vi "optimise_BBO_position.vi"(0 "Laser Power Q":T2, 7 "Controls Cluster":T1 {"Initial Step Direction" items=["Negative", "Positive"]}, 11 "error in (no error)":errorcluster) -> (8 "Optimised BBO crystal position":i32, 15 "error out":errorcluster)   [LabVIEW 2023]
panel:
  in  "stop":bool
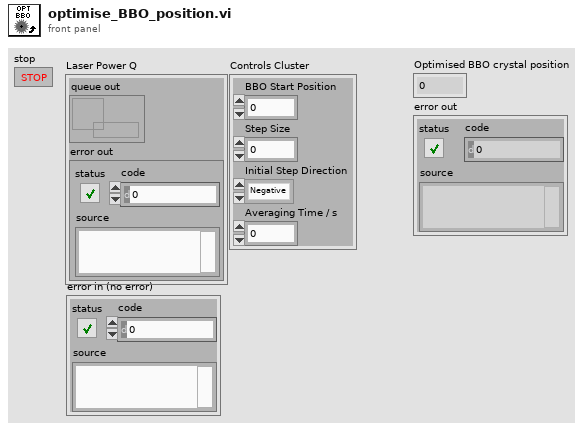
[diagram p1: front panel]
types:
  T1 = cluster{"BBO Start Position":i32, "Step Size":i32, "Initial Step Direction":u16, "Averaging Time / s ":u32}
  T2 = cluster{"queue out":refnum<queue>, "error out":errorcluster}
  T3 = cluster{"notifier out":refnum<notifier>, "error out":errorcluster}
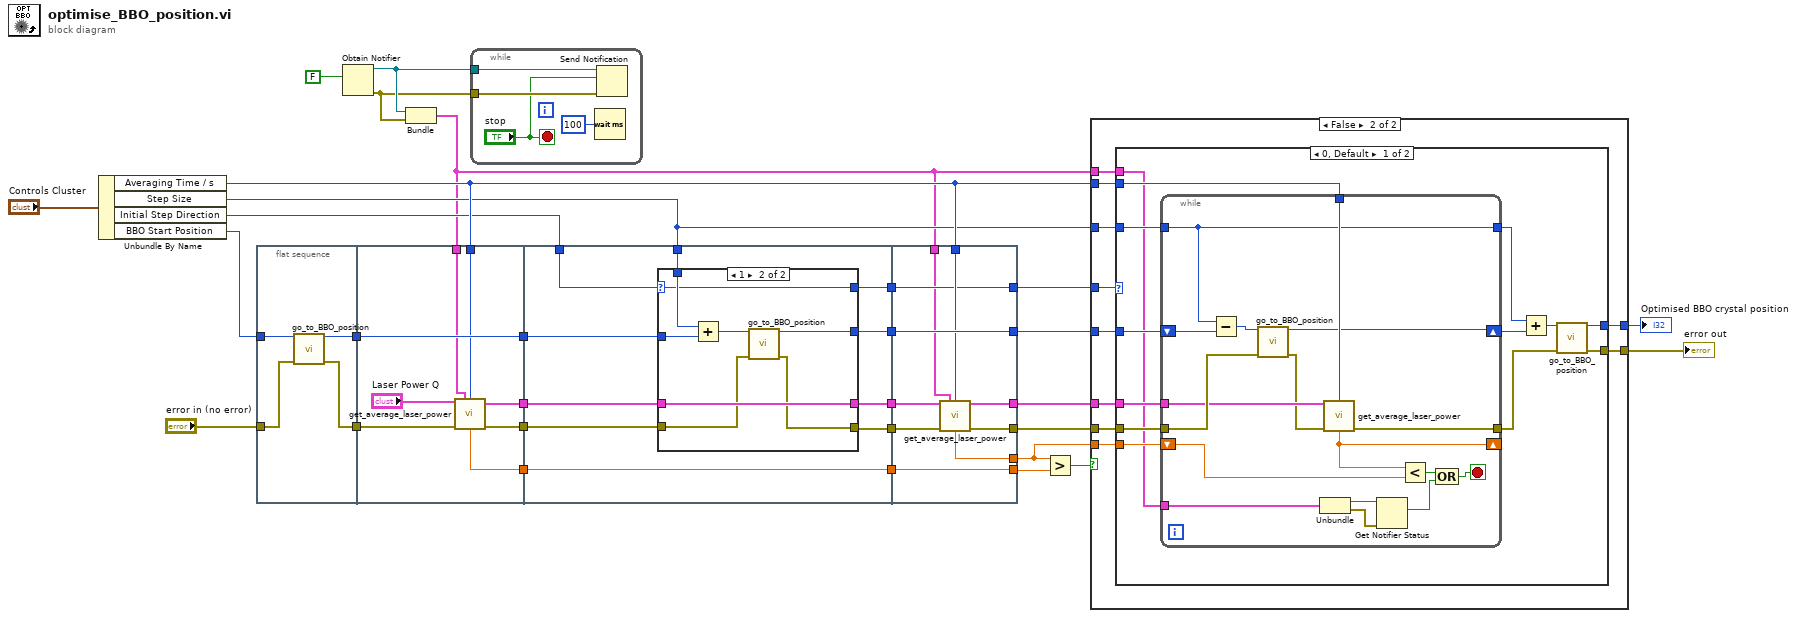
[diagram p0: block diagram]
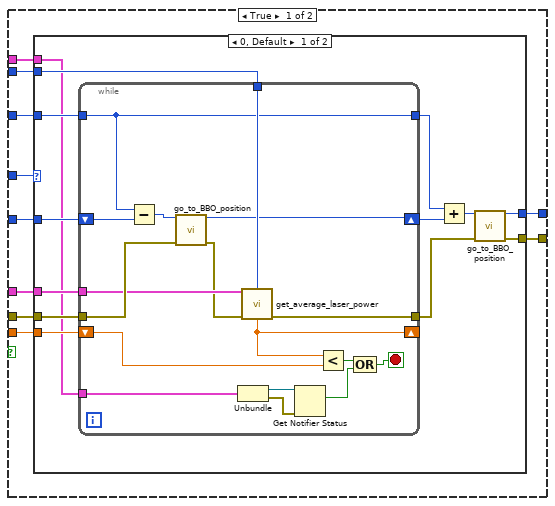
[diagram p2: hidden frame]
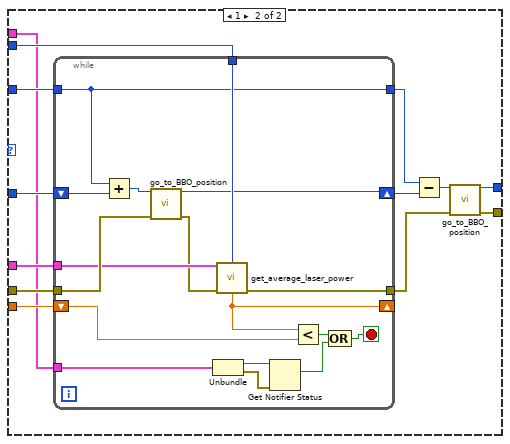
[diagram p3: hidden frame]
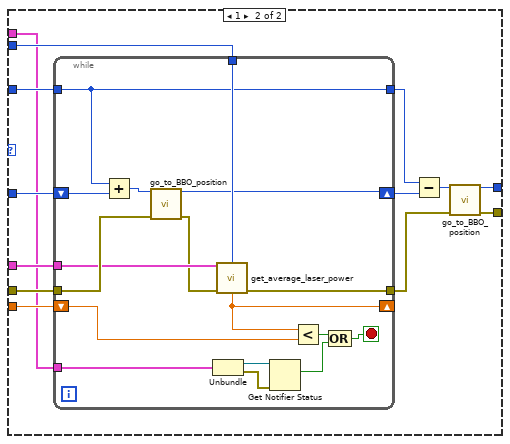
[diagram p4: hidden frame]
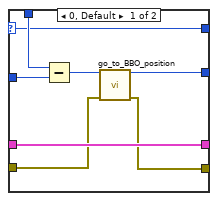
[diagram p5: hidden frame]
diagram:
  n1 = Unbundle By Name("Controls Cluster") -> ("Averaging Time / s"=w8:u32, "Step Size"=w6:i32, "Initial Step Direction"=w5:u16, "BBO Start Position"=w7:i32)
  n2 = flat-sequence {
    tunnel: w7 -> [w34]
    tunnel: "error in (no error)" -> [w33]
    tunnel: [w32] -> w29
    tunnel: [w31] -> w28
    tunnel: w29 -> [w42]
    tunnel: w28 -> [w37]
    tunnel: [w41] -> w27
    tunnel: [w40] -> w26
    tunnel: [w38] -> w25
    tunnel: [w37] -> w24
    tunnel: w8 -> [w36]
    tunnel: w1 -> [w35]
    tunnel: w27 -> [w50]
    tunnel: w26 -> [w45]
    tunnel: w25 -> [w51]
    tunnel: w24 -> [w49]
    tunnel: w6 -> [w52]
    tunnel: [w48] -> w23
    tunnel: [w47] -> w22
    tunnel: [w46] -> w21
    tunnel: [w45] -> w20
    tunnel: [w44] -> w14
    tunnel: w5 -> [w43]
    tunnel: w23 -> [w78]
    tunnel: w22 -> [w77]
    tunnel: w21 -> [w76]
    tunnel: w8 -> [w73]
    tunnel: w20 -> [w71]
    tunnel: [w78] -> w17
    tunnel: [w75] -> w16
    tunnel: [w74] -> w15
    tunnel: [w72] -> w12
    tunnel: [w71] -> w19
    tunnel: w14 -> [w70]
    tunnel: [w70] -> w13
    tunnel: w1 -> [w69]
    frame #0 {
      n3 = call "go_to_BBO_position.vi"("Set BBO crystal position"=w34, "error in (no error)"=w33) -> ("BBO crystal position"=w31:i32, "error out"=w32:errorcluster)  [unwired: 11 in, 1 out]
    }
    frame #1 {
      n4 = call "get_average_laser_power.vi"("Laser Power Q"="Laser Power Q", "Cancel Notifier"=w35, "Averaging Time /s"=w36, "Error in"=w42) -> ("Laser Power Q Out"=w38:T2, "Average Power / J"=w40:dbl, "Error out"=w41:errorcluster)  [unwired: 9 in]
    }
    frame #2 {
      n5 = case shown="1" w43 {
        selector: w43 -> [w53 w61]
        tunnel: w52 -> [w56 w64]
        tunnel: w51 -> [w60 w68]
        tunnel: [w60 w68] -> w47
        tunnel: w50 -> [w59 w67]
        tunnel: [w58 w66] -> w46
        tunnel: w49 -> [w55 w63]
        tunnel: [w54 w62] -> w48
        tunnel: [w53 w61] -> w44
        frame 0, Default {
          n6 = Subtract(x=w56, y=w55) -> (x-y=w57:i32)
          n7 = call "go_to_BBO_position.vi"("Set BBO crystal position"=w57, "error in (no error)"=w59) -> ("BBO crystal position"=w54:i32, "error out"=w58:errorcluster)  [unwired: 11 in, 1 out]
        }
        frame 1 {
          n8 = Add(x=w64, y=w63) -> (x+y=w65:i32)
          n9 = call "go_to_BBO_position.vi"("Set BBO crystal position"=w65, "error in (no error)"=w67) -> ("BBO crystal position"=w62:i32, "error out"=w66:errorcluster)  [unwired: 11 in, 1 out]
        }
      }
    }
    frame #3 {
      n10 = call "get_average_laser_power.vi"("Laser Power Q"=w77, "Cancel Notifier"=w69, "Averaging Time /s"=w73, "Error in"=w76) -> ("Laser Power Q Out"=w75:T2, "Average Power / J"=w72:dbl, "Error out"=w74:errorcluster)  [unwired: 9 in]
    }
  }
  n11 = Obtain Notifier(notification data type=FALSE ("stop")) -> (notifier out=w3:refnum<notifier>, error out=w2:errorcluster)  [unwired: 3 in, 1 out]
  n12 = Bundle("notifier out"=w3, "error out"=w2) -> (w1:T3)  [unwired: 1 in]
  n13 = while {
    tunnel: w3 -> [w81]
    tunnel: w2 -> [w80]
    stop <- "stop" stop-if-true
    n14 = Wait (ms)(milliseconds to wait=u32 100) -> ()  [unwired: 1 out]
    n15 = Send Notification(notification="stop", notifier=w81, error in (no error)=w80) -> ()  [unwired: 2 out]
  }
  n16 = Greater?(x=w12, y=w19) -> (0:w18:bool)
  n17 = case shown="False" w18 {
    tunnel: w17 -> [w91 w161]
    tunnel: w16 -> [w90 w160]
    tunnel: w15 -> [w89 w159]
    tunnel: w13 -> [w92 w162]
    tunnel: w6 -> [w88 w158]
    tunnel: w8 -> [w87 w157]
    tunnel: w12 -> [w86 w156]
    tunnel: [w85 w155] -> w11
    tunnel: [w84 w154] -> w10
    tunnel: w1 -> [w83 w153]
    frame True {
      n18 = case shown="0, Default" w92 {
        tunnel: w91 -> [w105 w135]
        tunnel: w90 -> [w104 w134]
        tunnel: w89 -> [w103 w133]
        tunnel: w88 -> [w102 w132]
        tunnel: w87 -> [w101 w131]
        tunnel: w86 -> [w100 w130]
        tunnel: [w95 w125] -> w85
        tunnel: [w94 w124] -> w84
        tunnel: w83 -> [w93 w123]
        frame 0, Default {
          n19 = while {
            tunnel: w104 -> [w119]
            tunnel: w103 -> [w122]
            tunnel: w102 -> [w112]
            tunnel: [w117] -> w96
            tunnel: w101 -> [w116]
            shift-right: [w115] -> w99
            shift-left: w105 -> [w120]
            shift-right: [w114] -> _
            shift-left: w100 -> [w113]
            tunnel: [w112] -> w98
            tunnel: w93 -> [w111]
            stop <- w108 stop-if-true
            n20 = Subtract(x=w112, y=w120) -> (x-y=w121:i32)
            n21 = call "go_to_BBO_position.vi"("Set BBO crystal position"=w121, "error in (no error)"=w122) -> ("BBO crystal position"=w115:i32, "error out"=w118:errorcluster)  [unwired: 11 in, 1 out]
            n22 = Unbundle(w111) -> ("notifier out"=w110:refnum<notifier>, "error out"=w109:errorcluster)
            n23 = call "get_average_laser_power.vi"("Laser Power Q"=w119, "Averaging Time /s"=w116, "Error in"=w118) -> ("Average Power / J"=w114:dbl, "Error out"=w117:errorcluster)  [unwired: 10 in, 1 out]
            n24 = Get Notifier Status(notifier=w110, error in (no error)=w109) -> (current notification=w106:bool)  [unwired: 4 out]
            n25 = Less?(x=w114, y=w113) -> (x < y?=w107:bool)
            n26 = Compound Arithmetic op=OR(w107, w106) -> (w108:bool)
          }
          n27 = Add(x=w98, y=w99) -> (x+y=w97:i32)
          n28 = call "go_to_BBO_position.vi"("Set BBO crystal position"=w97, "error in (no error)"=w96) -> ("BBO crystal position"=w95:i32, "error out"=w94:errorcluster)  [unwired: 11 in, 1 out]
        }
        frame 1 {
          n29 = while {
            tunnel: w134 -> [w149]
            tunnel: w133 -> [w152]
            tunnel: w132 -> [w142]
            tunnel: [w147] -> w126
            tunnel: w131 -> [w146]
            shift-right: [w145] -> w129
            shift-left: w135 -> [w150]
            shift-right: [w144] -> _
            shift-left: w130 -> [w143]
            tunnel: [w142] -> w128
            tunnel: w123 -> [w141]
            stop <- w138 stop-if-true
            n30 = Add(x=w142, y=w150) -> (x+y=w151:i32)
            n31 = call "go_to_BBO_position.vi"("Set BBO crystal position"=w151, "error in (no error)"=w152) -> ("BBO crystal position"=w145:i32, "error out"=w148:errorcluster)  [unwired: 11 in, 1 out]
            n32 = Unbundle(w141) -> ("notifier out"=w140:refnum<notifier>, "error out"=w139:errorcluster)
            n33 = call "get_average_laser_power.vi"("Laser Power Q"=w149, "Averaging Time /s"=w146, "Error in"=w148) -> ("Average Power / J"=w144:dbl, "Error out"=w147:errorcluster)  [unwired: 10 in, 1 out]
            n34 = Get Notifier Status(notifier=w140, error in (no error)=w139) -> (current notification=w136:bool)  [unwired: 4 out]
            n35 = Less?(x=w144, y=w143) -> (x < y?=w137:bool)
            n36 = Compound Arithmetic op=OR(w137, w136) -> (w138:bool)
          }
          n37 = Subtract(x=w128, y=w129) -> (x-y=w127:i32)
          n38 = call "go_to_BBO_position.vi"("Set BBO crystal position"=w127, "error in (no error)"=w126) -> ("BBO crystal position"=w125:i32, "error out"=w124:errorcluster)  [unwired: 11 in, 1 out]
        }
      }
    }
    frame False {
      n39 = case shown="0, Default" w162 {
        tunnel: w161 -> [w175 w205]
        tunnel: w160 -> [w174 w204]
        tunnel: w159 -> [w173 w203]
        tunnel: w158 -> [w172 w202]
        tunnel: w157 -> [w171 w201]
        tunnel: w156 -> [w170 w200]
        tunnel: [w165 w195] -> w155
        tunnel: [w164 w194] -> w154
        tunnel: w153 -> [w163 w193]
        frame 0, Default {
          n40 = while {
            tunnel: w174 -> [w189]
            tunnel: w173 -> [w192]
            tunnel: w172 -> [w182]
            tunnel: [w187] -> w166
            tunnel: w171 -> [w186]
            shift-right: [w185] -> w169
            shift-left: w175 -> [w190]
            shift-right: [w184] -> _
            shift-left: w170 -> [w183]
            tunnel: [w182] -> w168
            tunnel: w163 -> [w181]
            stop <- w178 stop-if-true
            n41 = Subtract(x=w182, y=w190) -> (x-y=w191:i32)
            n42 = call "go_to_BBO_position.vi"("Set BBO crystal position"=w191, "error in (no error)"=w192) -> ("BBO crystal position"=w185:i32, "error out"=w188:errorcluster)  [unwired: 11 in, 1 out]
            n43 = Unbundle(w181) -> ("notifier out"=w180:refnum<notifier>, "error out"=w179:errorcluster)
            n44 = call "get_average_laser_power.vi"("Laser Power Q"=w189, "Averaging Time /s"=w186, "Error in"=w188) -> ("Average Power / J"=w184:dbl, "Error out"=w187:errorcluster)  [unwired: 10 in, 1 out]
            n45 = Get Notifier Status(notifier=w180, error in (no error)=w179) -> (current notification=w176:bool)  [unwired: 4 out]
            n46 = Less?(x=w184, y=w183) -> (x < y?=w177:bool)
            n47 = Compound Arithmetic op=OR(w177, w176) -> (w178:bool)
          }
          n48 = Add(x=w168, y=w169) -> (x+y=w167:i32)
          n49 = call "go_to_BBO_position.vi"("Set BBO crystal position"=w167, "error in (no error)"=w166) -> ("BBO crystal position"=w165:i32, "error out"=w164:errorcluster)  [unwired: 11 in, 1 out]
        }
        frame 1 {
          n50 = while {
            tunnel: w204 -> [w219]
            tunnel: w203 -> [w222]
            tunnel: w202 -> [w212]
            tunnel: [w217] -> w196
            tunnel: w201 -> [w216]
            shift-right: [w215] -> w199
            shift-left: w205 -> [w220]
            shift-right: [w214] -> _
            shift-left: w200 -> [w213]
            tunnel: [w212] -> w198
            tunnel: w193 -> [w211]
            stop <- w208 stop-if-true
            n51 = Add(x=w212, y=w220) -> (x+y=w221:i32)
            n52 = call "go_to_BBO_position.vi"("Set BBO crystal position"=w221, "error in (no error)"=w222) -> ("BBO crystal position"=w215:i32, "error out"=w218:errorcluster)  [unwired: 11 in, 1 out]
            n53 = Unbundle(w211) -> ("notifier out"=w210:refnum<notifier>, "error out"=w209:errorcluster)
            n54 = call "get_average_laser_power.vi"("Laser Power Q"=w219, "Averaging Time /s"=w216, "Error in"=w218) -> ("Average Power / J"=w214:dbl, "Error out"=w217:errorcluster)  [unwired: 10 in, 1 out]
            n55 = Get Notifier Status(notifier=w210, error in (no error)=w209) -> (current notification=w206:bool)  [unwired: 4 out]
            n56 = Less?(x=w214, y=w213) -> (x < y?=w207:bool)
            n57 = Compound Arithmetic op=OR(w207, w206) -> (w208:bool)
          }
          n58 = Subtract(x=w198, y=w199) -> (x-y=w197:i32)
          n59 = call "go_to_BBO_position.vi"("Set BBO crystal position"=w197, "error in (no error)"=w196) -> ("BBO crystal position"=w195:i32, "error out"=w194:errorcluster)  [unwired: 11 in, 1 out]
        }
      }
    }
  }
  "Optimised BBO crystal position" <- w11
  "error out" <- w10
